vi "Create Plot Object.vi"(6 "Control Ref Queue":T1, 7 "Actual Transform In":T2, 8 "error in (no error)":errorcluster, 9 "Multiplot Representation In":T4, 10 "3D Plot.lvclass in":refnum<class "3D Plot.lvclass">, 11 "Plot Object In":refnum<vi>) -> (0 "error out":errorcluster, 1 "Multiplot Representation Out":T4, 2 "3D Plot.lvclass out":refnum<class "3D Plot.lvclass">, 3 "Plot Object Out":refnum<vi>, 5 "Actual Transform Out":T2)   [LabVIEW 2017, in "3D Plot.lvclass"]
uses:
  <vilib>/Math Plots/3D Math Plots/3D Plot/3D Plot/3D Plot.lvclass
  <vilib>/Math Plots/3D Math Plots/3D Plot/3D Plot/Typedef/Multiplot Representation.ctl
  <vilib>/Math Plots/3D Math Plots/3D Plot/3D Plot/Typedef/Plot Representation.ctl
  <vilib>/Math Plots/3D Math Plots/3D Plot/3D Plot/Typedef/Range Clusters.ctl
  <vilib>/Math Plots/3D Math Plots/3D Plot/3D Plot/Typedef/Mesh Data.ctl
  <vilib>/Math Plots/3D Math Plots/3D Plot/3D Plot/Typedef/Actual Transform.ctl
  <vilib>/Math Plots/3D Math Plots/3D Plot/Action String/3DMathPlot Ctrl Act Queue.ctl
  <vilib>/Math Plots/3D Math Plots/3D Plot/Action String/3DMathPlot Ctrl Act Cluster.ctl
  <vilib>/Math Plots/3D Math Plots/3D Plot/Action String/3DMathPlot State Class.ctl
  <vilib>/Math Plots/3D Math Plots/3D Plot/3D Plot/3D Plot.lvclass/3D Plot.ctl
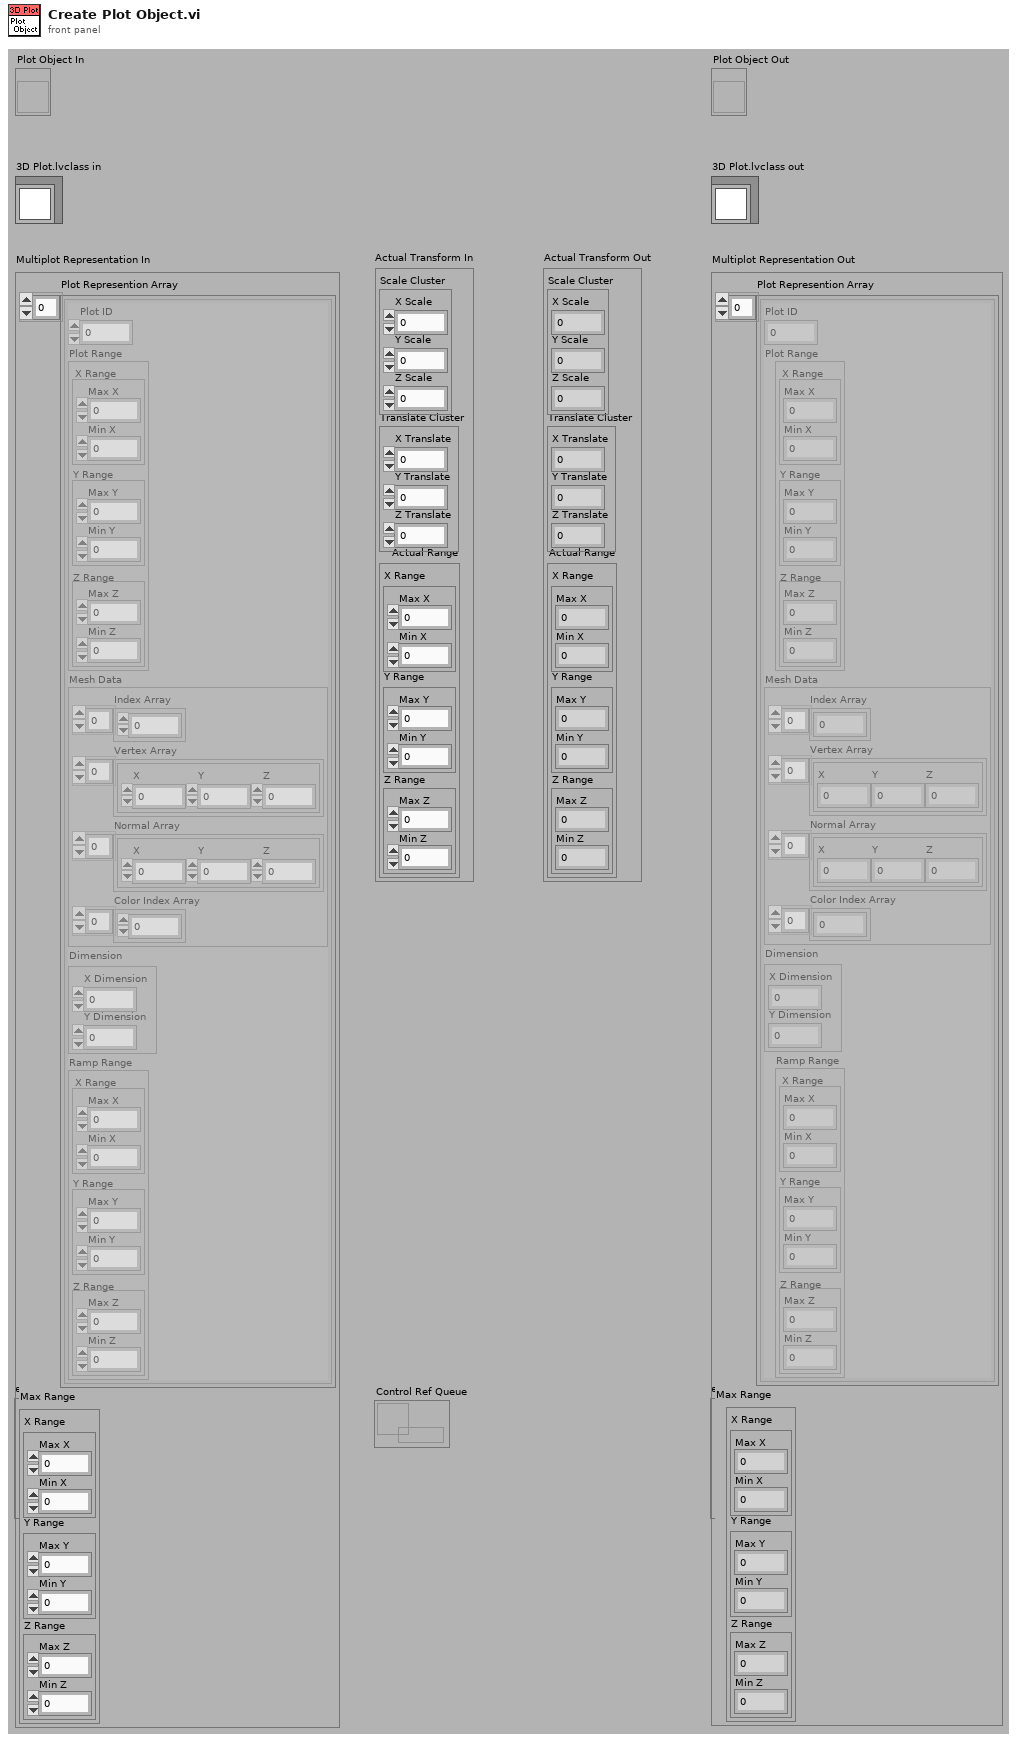
[diagram p1: front panel]
types:
  T1 = typedef "3DMathPlot Ctrl Act Queue.ctl" = refnum<queue>
  T2 = typedef "3D Plot.lvclass/Actual Transform.ctl" = cluster{"Scale Cluster":cluster{"X Scale":sgl, "Y Scale":sgl, "Z Scale":sgl}, "Translate Cluster":cluster{"X Translate":sgl, "Y Translate":sgl, "Z Translate":sgl}, "Actual Range":T3}
  T3 = typedef "3D Plot.lvclass/Range Clusters.ctl" = cluster{"X Range":cluster{"Max X":sgl, "Min X":sgl}, "Y Range":cluster{"Max Y":sgl, "Min Y":sgl}, "Z Range":cluster{"Max Z":sgl, "Min Z":sgl}}
  T4 = typedef "3D Plot.lvclass/Multiplot Representation.ctl" = cluster{"Plot Represention Array":T5[], "Max Range":T3}
  T5 = typedef "3D Plot.lvclass/Plot Representation.ctl" = cluster{"Plot ID":i32, "Plot Range":T3, "Mesh Data":T6, "Dimension":cluster{"X Dimension":i32, "Y Dimension":i32}, "Ramp Range":T3}
  T6 = typedef "3D Plot.lvclass/Mesh Data.ctl" = cluster{"Index Array":u32[], "Vertex Array":cluster{"X":sgl, "Y":sgl, "Z":sgl}[], "Normal Array":cluster{"X":sgl, "Y":sgl, "Z":sgl}[], "Color Index Array":i32[]}
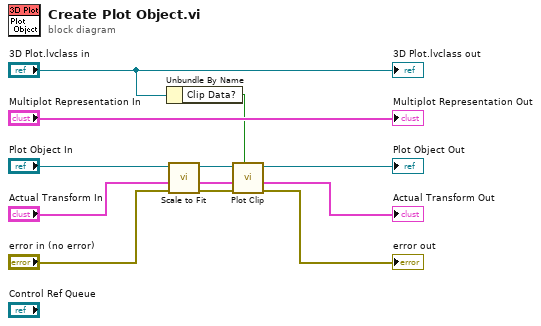
[diagram p0: block diagram]
diagram:
  n1 = Unbundle By Name("3D Plot.lvclass in") -> ("Clip Data?"=w6:bool)
  n2 = call <vilib>:"Scale to Fit.vi"("error in (no error)"="error in (no error)", "Actual Transform In"="Actual Transform In", "Plot Object In"="Plot Object In") -> ("error out"=w3:errorcluster, "Actual Transform Out"=w4:T2, "Plot Object Out"=w5:refnum<vi>)  [unwired: 6 out]
  n3 = call <vilib>:"Plot Clip.vi"("Clip Data"=w6, "error in (no error)"=w3, "Actual Transform In"=w4, "Plot Object In"=w5) -> ("error out"=→"error out":errorcluster, "Actual Transform Out"=→"Actual Transform Out":T2, "Plot Object Out"=→"Plot Object Out":refnum<vi>)  [unwired: 5 out]
  "3D Plot.lvclass out" <- "3D Plot.lvclass in"
  "Multiplot Representation Out" <- "Multiplot Representation In"
